vi "20220713 PI comm test.vi"() -> ()   [LabVIEW 2020]
uses:
  <vilib>/Instr/_visa.llb/VISA Configure Serial Port (Instr).vi
panel:
  in  "Func delay input":dbl caption="0.01 - 1 s"
  in  "Func on Time input":dbl caption="0.01 - 1 s"
  in  "Func freq input":dbl caption="10 - 10k Hz"
  in  "Func amp input":dbl caption="0 - 5 V"
  in  "PMT2 senstivity input":dbl caption="0.5-0.75 V"
  in  "PMT1 senstivity input":dbl caption="0.5-0.75 V"
  in  "Func Delay":bool
  in  "Func On time":bool
  in  "Func Freq":bool
  in  "Func amp":bool
  in  "PMT2 senstivity":bool
  in  "PMT1 senstivity":bool
  out "read":string
  in  "Initializer":bool
  in  "Shut down program":bool=TRUE
  in  "COM port number":refnum<visa-resource-name>="COM8"
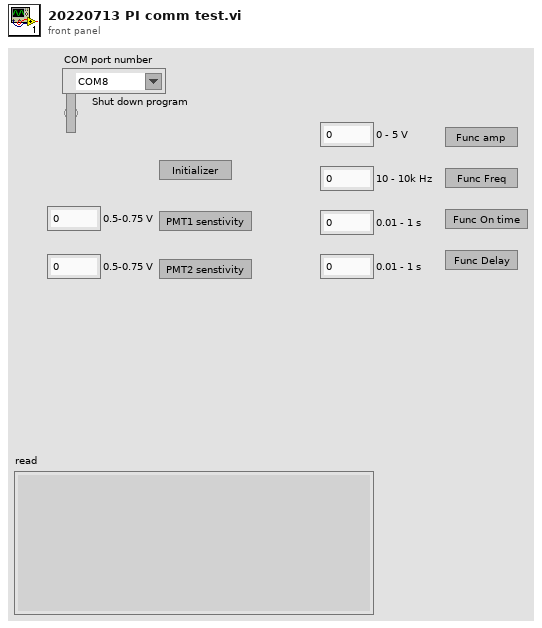
[diagram p1: front panel]
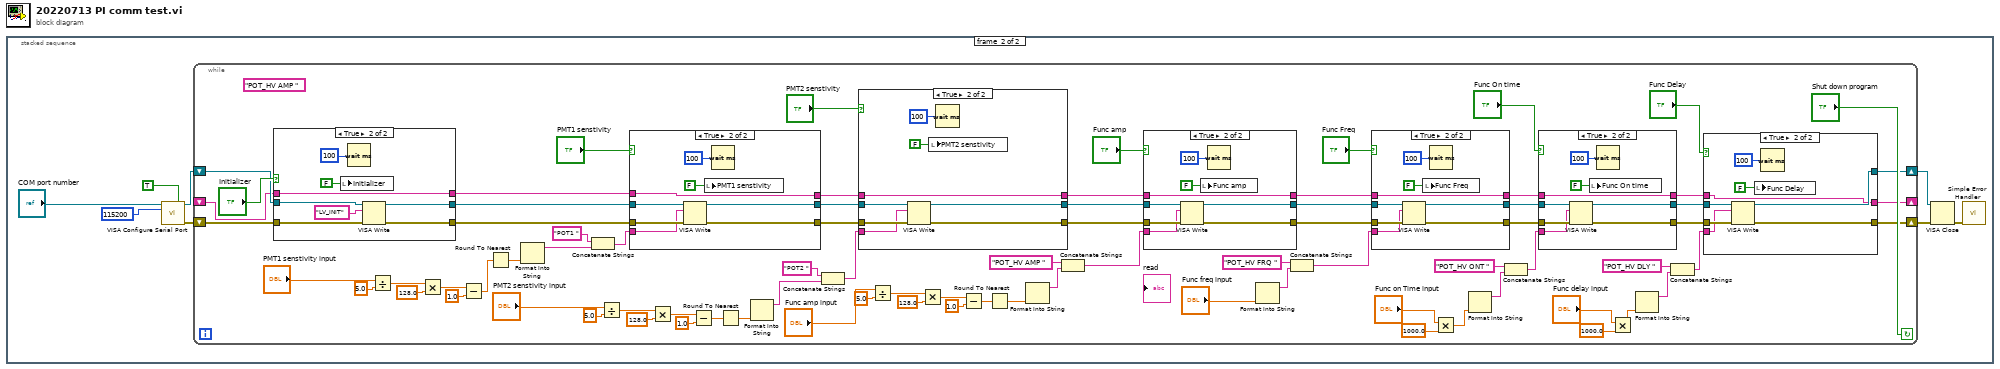
[diagram p0: block diagram]
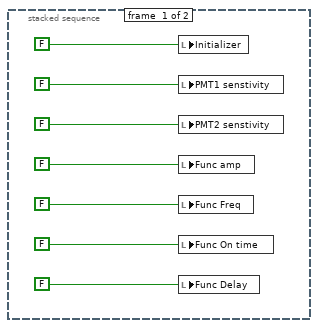
[diagram p2: hidden frame]
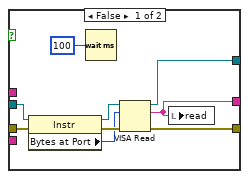
[diagram p3: hidden frame]
diagram:
  n1 = stacked-sequence {
    frame #0 {
      n2 = local write "Initializer"(FALSE ("send")) -> ()
      n3 = local write "PMT1 senstivity"(FALSE ("send")) -> ()
      n4 = local write "PMT2 senstivity"(FALSE ("send")) -> ()
      n5 = local write "Func amp"(FALSE ("send")) -> ()
      n6 = local write "Func Freq"(FALSE ("send")) -> ()
      n7 = local write "Func On time"(FALSE ("send")) -> ()
      n8 = local write "Func Delay"(FALSE ("send")) -> ()
    }
    frame #1 {
      n9 = call-poly "VISA Configure Serial Port"("VISA resource name"="COM port number", "Enable Termination\nChar (T)"=TRUE ("Enable Termination\nChar (T)"), "baud rate (9600)"=u32 115200) -> ("VISA resource name out"=w11:refnum<visa-resource-name>, "error out"=w10:errorcluster)  [unwired: 11 in]
      n10 = while {
        shift-right: [w75] -> w8
        shift-left: w11 -> [w95]
        shift-right: [w74] -> w12
        shift-left: w10 -> [w94]
        shift-right: [w76] -> _
        shift-left: _ -> [w92]
        stop <- "Shut down program" continue-if-true
        (unwired) "POT_HV AMP " ("string")
        n11 = case shown="True" "Initializer" {
          tunnel: w95 -> [w169 w179]
          tunnel: w94 -> [w170 w178]
          tunnel: [w169 w175] -> w91
          tunnel: [w170 w174] -> w90
          tunnel: w92 -> [w171 w173]
          tunnel: [w171 w173] -> w89
          frame False {
          }
          frame True {
            n12 = local write "Initializer"(FALSE ("send")) -> ()
            n13 = Wait (ms)(milliseconds to wait=u32 100) -> ()  [unwired: 1 out]
            n14 = VISA Write(VISA resource name=w179, write buffer="LV_INIT", error in (no error)=w178) -> (VISA resource name out=w175:refnum<visa-resource-name>, error out=w174:errorcluster)  [unwired: 1 out]
          }
        }
        n15 = Divide(x="PMT1 senstivity input", y=5.0) -> (x/y=w58:dbl)
        n16 = Multiply(x=w58, y=128.0) -> (x*y=w60:dbl)
        n17 = Subtract(x=w60, y=1.0) -> (x-y=w55:dbl)
        n18 = Round To Nearest(number=w55) -> (nearest integer value=w64:dbl)
        n19 = Format Into String(w64) -> (resulting string=w63:string)  [unwired: 3 in, 1 out]
        n20 = Concatenate Strings("POT1 " ("string"), w63) -> (w61:string)
        n21 = Divide(x="PMT2 senstivity input", y=5.0) -> (x/y=w50:dbl)
        n22 = case shown="True" "PMT1 senstivity" {
          tunnel: w91 -> [w159 w168]
          tunnel: w90 -> [w158 w167]
          tunnel: [w159 w164] -> w88
          tunnel: [w158 w163] -> w87
          tunnel: w89 -> [w160 w162]
          tunnel: [w160 w162] -> w86
          tunnel: w61 -> [_ w161]
          frame False {
          }
          frame True {
            n23 = VISA Write(VISA resource name=w168, write buffer=w161, error in (no error)=w167) -> (VISA resource name out=w164:refnum<visa-resource-name>, error out=w163:errorcluster)  [unwired: 1 out]
            n24 = local write "PMT1 senstivity"(FALSE ("send")) -> ()
            n25 = Wait (ms)(milliseconds to wait=u32 100) -> ()  [unwired: 1 out]
          }
        }
        n26 = Multiply(x=w50, y=128.0) -> (x*y=w48:dbl)
        n27 = Subtract(x=w48, y=1.0) -> (x-y=w52:dbl)
        n28 = Round To Nearest(number=w52) -> (nearest integer value=w45:dbl)
        n29 = Format Into String(w45) -> (resulting string=w46:string)  [unwired: 3 in, 1 out]
        n30 = Concatenate Strings("POT2 " ("string"), w46) -> (w43:string)
        n31 = case shown="True" "PMT2 senstivity" {
          tunnel: w88 -> [w147 w157]
          tunnel: w87 -> [w148 w156]
          tunnel: [w147 w153] -> w72
          tunnel: [w148 w152] -> w71
          tunnel: w86 -> [w149 w151]
          tunnel: [w149 w151] -> w73
          tunnel: w43 -> [_ w150]
          frame False {
          }
          frame True {
            n32 = VISA Write(VISA resource name=w157, write buffer=w150, error in (no error)=w156) -> (VISA resource name out=w153:refnum<visa-resource-name>, error out=w152:errorcluster)  [unwired: 1 out]
            n33 = local write "PMT2 senstivity"(FALSE ("send")) -> ()
            n34 = Wait (ms)(milliseconds to wait=u32 100) -> ()  [unwired: 1 out]
          }
        }
        n35 = Divide(x="Func amp input", y=5.0) -> (x/y=w37:dbl)
        n36 = Multiply(x=w37, y=128.0) -> (x*y=w39:dbl)
        n37 = Subtract(x=w39, y=1.0) -> (x-y=w35:dbl)
        n38 = Round To Nearest(number=w35) -> (nearest integer value=w41:dbl)
        n39 = Format Into String(w41) -> (resulting string=w40:string)  [unwired: 3 in, 1 out]
        n40 = Concatenate Strings("POT_HV AMP " ("string"), w40) -> (w33:string)
        n41 = case shown="True" "Func amp" {
          tunnel: w72 -> [w138 w146]
          tunnel: w71 -> [w136 w145]
          tunnel: [w138 w142] -> w85
          tunnel: [w136 w141] -> w84
          tunnel: w73 -> [w137 w140]
          tunnel: [w137 w140] -> w83
          tunnel: w33 -> [_ w139]
          frame False {
          }
          frame True {
            n42 = VISA Write(VISA resource name=w146, write buffer=w139, error in (no error)=w145) -> (VISA resource name out=w142:refnum<visa-resource-name>, error out=w141:errorcluster)  [unwired: 1 out]
            n43 = local write "Func amp"(FALSE ("send")) -> ()
            n44 = Wait (ms)(milliseconds to wait=u32 100) -> ()  [unwired: 1 out]
          }
        }
        n45 = Format Into String("Func freq input") -> (resulting string=w32:string)  [unwired: 3 in, 1 out]
        n46 = Concatenate Strings("POT_HV FRQ " ("string"), w32) -> (w29:string)
        n47 = case shown="True" "Func Freq" {
          tunnel: w85 -> [w126 w135]
          tunnel: w84 -> [w125 w134]
          tunnel: [w126 w131] -> w77
          tunnel: [w125 w130] -> w78
          tunnel: w83 -> [w127 w129]
          tunnel: [w127 w129] -> w82
          tunnel: w29 -> [_ w128]
          frame False {
          }
          frame True {
            n48 = VISA Write(VISA resource name=w135, write buffer=w128, error in (no error)=w134) -> (VISA resource name out=w131:refnum<visa-resource-name>, error out=w130:errorcluster)  [unwired: 1 out]
            n49 = local write "Func Freq"(FALSE ("send")) -> ()
            n50 = Wait (ms)(milliseconds to wait=u32 100) -> ()  [unwired: 1 out]
          }
        }
        n51 = Multiply(x="Func on Time input", y=1000.0) -> (x*y=w19:dbl)
        n52 = Format Into String(w19) -> (resulting string=w28:string)  [unwired: 3 in, 1 out]
        n53 = Concatenate Strings("POT_HV ONT " ("string"), w28) -> (w27:string)
        n54 = case shown="True" "Func On time" {
          tunnel: w78 -> [w114 w124]
          tunnel: [w115 w121] -> w80
          tunnel: [w114 w120] -> w79
          tunnel: w82 -> [w116 w119]
          tunnel: [w116 w119] -> w81
          tunnel: w77 -> [w115 w118]
          tunnel: w27 -> [_ w117]
          frame False {
          }
          frame True {
            n55 = VISA Write(VISA resource name=w118, write buffer=w117, error in (no error)=w124) -> (VISA resource name out=w121:refnum<visa-resource-name>, error out=w120:errorcluster)  [unwired: 1 out]
            n56 = local write "Func On time"(FALSE ("send")) -> ()
            n57 = Wait (ms)(milliseconds to wait=u32 100) -> ()  [unwired: 1 out]
          }
        }
        n58 = Multiply(x="Func delay input", y=1000.0) -> (x*y=w17:dbl)
        n59 = Format Into String(w17) -> (resulting string=w26:string)  [unwired: 3 in, 1 out]
        n60 = Concatenate Strings("POT_HV DLY " ("string"), w26) -> (w25:string)
        n61 = case shown="True" "Func Delay" {
          tunnel: w80 -> [w102 w113]
          tunnel: w79 -> [w101 w112]
          tunnel: [w100 w109] -> w75
          tunnel: [w99 w108] -> w74
          tunnel: w81 -> [_ w107]
          tunnel: [w97 w107] -> w76
          tunnel: w25 -> [_ w106]
          frame False {
            n62 = property class="Instr"(reference=w102, error in=w101) -> (reference out=w103:refnum<visa-resource-name>, error out=w105:errorcluster, "Bytes at Port"=w104:u32)
            n63 = Wait (ms)(milliseconds to wait=u32 100) -> ()  [unwired: 1 out]
            n64 = VISA Read(VISA resource name=w103, byte count=w104, error in (no error)=w105) -> (VISA resource name out=w100:refnum<visa-resource-name>, read buffer=w97:string, error out=w99:errorcluster)  [unwired: 1 out]
            n65 = local write "read"(w97) -> ()
          }
          frame True {
            n66 = VISA Write(VISA resource name=w113, write buffer=w106, error in (no error)=w112) -> (VISA resource name out=w109:refnum<visa-resource-name>, error out=w108:errorcluster)  [unwired: 1 out]
            n67 = local write "Func Delay"(FALSE ("send")) -> ()
            n68 = Wait (ms)(milliseconds to wait=u32 100) -> ()  [unwired: 1 out]
          }
        }
      }
      n69 = VISA Close(VISA resource name=w8, error in (no error)=w12) -> (error out=w13:errorcluster)
      n70 = call <vilib>:"Simple Error Handler.vi"("error in (no error)"=w13) -> ()  [unwired: 4 in, 5 out]
    }
  }
